vi "doAoWrite.vi"(8 "error in":errorcluster, 10 "Control Data":T1, 11 "DAQmx Container In":T2) -> (0 "error out":errorcluster, 2 "Control Data":T1, 3 "DAQmx Container Out":T2)   [LabVIEW 2024]
uses:
  support/Control/DAQmx Container.ctl
  support/Control/Control Data Constant.ctl
  <vilib>/DAQmx/write.llb/DAQmx Write (Digital 1D Bool NChan 1Samp 1Line).vi
  <vilib>/DAQmx/miscellaneous.llb/DAQmx Fill In Error Info.vi
  <resource>/objmgr/daqmx.rc
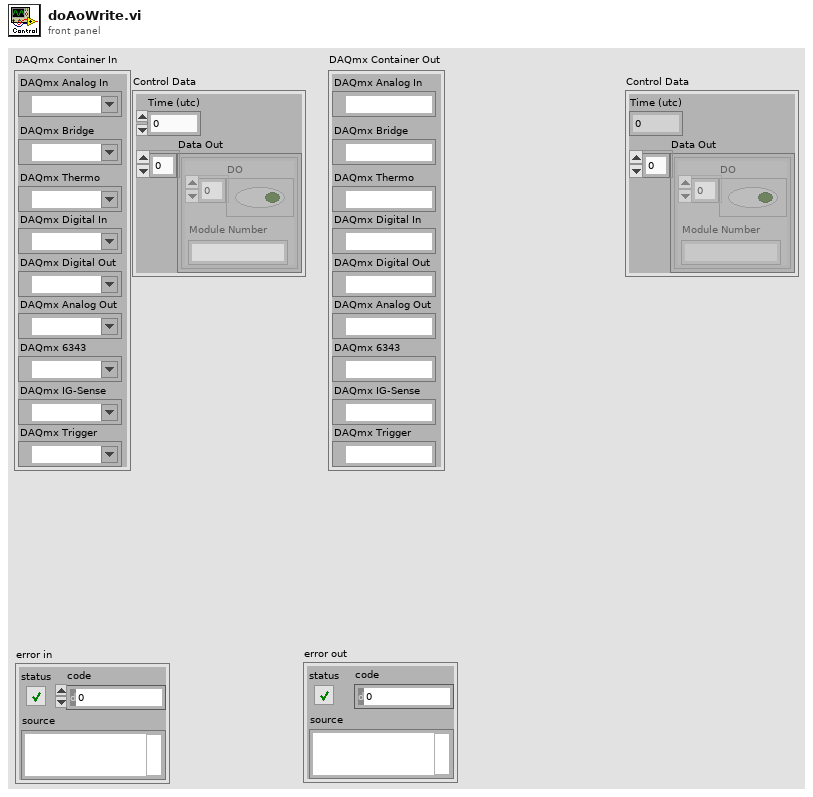
[diagram p1: front panel]
types:
  T1 = typedef "Control Data Constant.ctl" = cluster{"Time (utc)":ext, "Data Out":cluster{"DO":bool[], "Module Number":string}[]}
  T2 = typedef "DAQmx Container.ctl" = cluster{"DAQmx Analog In":refnum<k21>, "DAQmx Digital In":refnum<k21>, "DAQmx Digital Out":refnum<k21>, "DAQmx Analog Out":refnum<k21>, "DAQmx 6343":refnum<k21>, "DAQmx IG-Sense":refnum<k21>, "DAQmx Thermo":refnum<k21>, "DAQmx Bridge":refnum<k21>, "DAQmx Trigger":refnum<k21>}
  T3 = typedef "LVDateTimeRec.ctl" = cluster{"fractional second":dbl, "second":i32, "minute":i32, "hour":i32, "day of month":i32, "month":i32, "year":i32, "day of week":i32, "day of year":i32, "DST":i32}
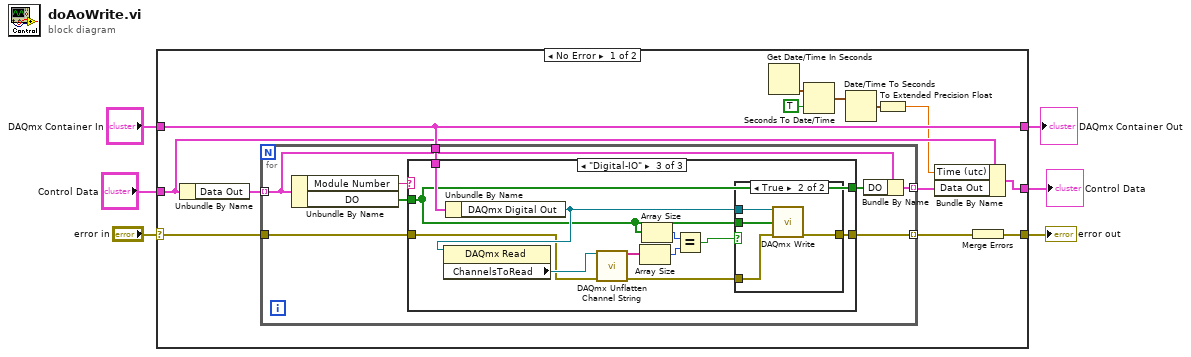
[diagram p0: block diagram]
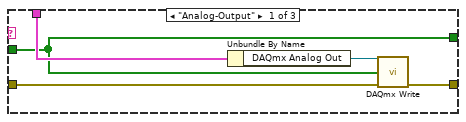
[diagram p2: hidden frame]
diagram:
  n1 = case shown="No Error" "error in" {
    selector: "error in" -> [w16 w53]
    tunnel: [w19 w53] -> w5
    tunnel: "DAQmx Container In" -> [w17 w52]
    tunnel: [w17 w52] -> w3
    tunnel: "Control Data" -> [w14 w51]
    tunnel: [w13 w51] -> w1
    frame No Error {
      n2 = Unbundle By Name(w14) -> ("Data Out"=w15:cluster{"DO":bool[], "Module Number":string}[])
      n3 = for {
        tunnel: [w27] -> w18 mode=indexing
        tunnel: w17 -> [w26]
        tunnel: w16 -> [w25]
        tunnel: [w23] -> w12 mode=indexing
        tunnel: w15 -> [w22] mode=indexing
        n4 = Unbundle By Name(w22) -> ("Module Number"=w24:string, "DO"=w21:bool[])
        n5 = case shown="\"Digital-IO\"" w24 {
          tunnel: [w32 w34 w35] -> w27
          tunnel: w26 -> [w30 _ w45]
          tunnel: w25 -> [w29 w34 w42]
          tunnel: w21 -> [w28 w33 w40]
          tunnel: [w28 w33 w40] -> w20
          frame "Analog-Output" {
            n6 = Unbundle By Name(w30) -> ("DAQmx Analog Out"=w31:refnum<k21>)
            n7 = call-poly <vilib>:"DAQmx Write.vi"("task/channels in"=w31, "data"=w28, "error in"=w29) -> ("error out"=w32:errorcluster)  [unwired: 10 in, 2 out]
          }
          frame Default {
          }
          frame "Digital-IO" {
            n8 = Unbundle By Name(w45) -> ("DAQmx Digital Out"=w44:refnum<k21>)
            n9 = property class="DAQmx Read"(reference=w44) -> ("ChannelsToRead"=w43:refnum<k21>)  [unwired: 1 in, 2 out]
            n10 = call <vilib>:"DAQmx Unflatten Channel String.vi"("names in"=w43, "error in"=w42) -> ("names out"=w41:string[], "error out"=w36:errorcluster)  [unwired: 12 in]
            n11 = Array Size(array=w41) -> (size(s)=w38:i32)
            n12 = Array Size(array=w40) -> (size(s)=w39:i32)
            n13 = Equal?(x=w39, y=w38) -> (x = y?=w37:bool)
            n14 = case shown="True" w37 {
              tunnel: w44 -> [_ w49]
              tunnel: w40 -> [_ w48]
              tunnel: w36 -> [w46 w47]
              tunnel: [w46 w50] -> w35
              frame False {
              }
              frame True {
                n15 = call-poly <vilib>:"DAQmx Write.vi"("task/channels in"=w49, "data"=w48, "error in"=w47) -> ("error out"=w50:errorcluster)  [unwired: 10 in, 2 out]
              }
            }
          }
        }
        n16 = Bundle By Name(cluster=w22, "DO"=w20) -> (w23:cluster{"DO":bool[], "Module Number":string})
      }
      n17 = Get Date/Time In Seconds() -> (seconds since 1Jan1904=w10:timestamp)
      n18 = Seconds To Date/Time(time stamp (now)=w10, to UTC (F)=TRUE) -> (date time rec=w11:T3)
      n19 = Date/Time To Seconds(2:w11) -> (0:w8:timestamp)  [unwired: 1 in]
      n20 = To Extended Precision Float(1:w8) -> (0:w7:ext)
      n21 = Bundle By Name(cluster=w14, "Time (utc)"=w7, "Data Out"=w12) -> (w13:T1)
      n22 = Merge Errors(w18) -> (w19:errorcluster)
    }
    frame Error {
    }
  }
  "error out" <- w5
  "DAQmx Container Out" <- w3
  "Control Data" <- w1
